vi "VelocityControl.vi"() -> ()   [LabVIEW 2024]
uses:
  <userlib>/SerialVIs/subs/portX.xctl
  <vilib>/Analysis/Matrix/Numeric/Multiply/Multiply - RM,R.vi
  <vilib>/Analysis/Matrix/Numeric/Add/Add - RM,RM.vi
  <vilib>/Analysis/Matrix/NI_Matrix.lvlib
panel:
  out "angles in deg":dbl[][](array[numeric])=[[-36.014154610778625, 83.46837607802595], [-30.58893000924773, 84.11552246158425], [-25.130229737371057, 84.75431124956516], [-19.634641879547157, 85.37840761378398], [-14.099111797871014, 85.98156827076336], [-8.52099033519902, 86.55769560527041], [-2.8980785837318344, 87.10089173956699], [2.7713319119854534, 87.60551252738216], [8.488424735842507, 88.06622131808514], [14.25383121793239, 88.47804217667414], [20.067611307066525, 88.83641207225367], [25.92924379518322, 89.13723137682419], [31.83762677661892, 89.37691186368073], [37.79108891767169, 89.55242127664737], [43.78741172147553, 89.66132347232612], [49.82386252120048, 89.70181312891611], [55.89723745208451, 89.67274407360235], [62.003913178065496, 89.57365040665448], [68.13990572321374, 89.40475978812653], [74.3009344212881, 89.16699848970453], [80.48248878103452, 88.86198808146582], [86.67989599134705, 88.4920338989176], [92.88838686585272, 88.06010569607713], [99.10315824254073, 87.5698111131883], [105.31943018881677, 87.02536275434173], [111.53249678363956, 86.43153976791783], [117.73776971827958, 85.79364484548083], [123.93081443693836, 85.11745750383476], [130.10737899266636, 84.40918439844886], [136.2634161940642, 83.67540724798543], [142.3950999438779, 82.92302874692331], [148.49883691016672, 82.15921662646399], [154.5712748202658, 81.39134581430122], [160.60930872926238, 80.62693846251224], [166.610086594057, 79.87360147972578], [172.57101538925974, 79.13896113671923], [178.4897688408234, 78.43059432862572], [184.36429763607669, 77.75595618282775], [190.1928427033293, 77.12230390469071], [195.97395184977762, 76.53661705157901], [201.7064997140921, 76.0055148080184], [207.38971064375187, 75.53517127963], [213.02318376462966, 75.131230297345], [218.6069191931086, 74.79872168252136], [224.14134407370238, 74.54198131618745], [229.62733693304716, 74.36457762732287], [235.06624874699818, 74.26924721603851], [240.45991913755014, 74.25784222094941], [245.81068625614293, 74.3312917102616], [251.12138916207132, 74.48957883430128], [256.39536184764745, 74.73173476319667], [261.6364184616579, 75.05584961216476], [266.8488296977405, 75.45909971015618], [272.0372907009237, 75.93778978209922], [277.20688116485434, 76.48740796901053], [282.3630185159317, 77.1026911624394], [287.5114051948649, 77.77769791154134], [292.65797105288704, 78.50588617461314], [297.80881179498004, 79.28019340777786], [302.9701242527187, 80.09311686760488], [308.1481390877215, 80.9367924966783], [313.3490513478763, 81.8030713039308], [318.5789491549387, 82.68359269188973]]
  out "End eff positions":dbl[][](array[numeric])=[[118.80406614490178, 11.900177338584307], [116.42319949227772, 23.62061939757193], [112.8812852219431, 35.0439304341559], [108.21380153738838, 46.05570065265972], [102.46745978970496, 56.545646687002716], [95.69973332672421, 66.40870931198523], [87.97828022716507, 75.54609771369901], [79.38026604839743, 83.86627031856675], [69.99159358054067, 91.28584292437694], [59.90604735660835, 97.73041567276096], [49.22436132278885, 103.13531122901531], [38.05321863612864, 107.44621737344505], [26.50419304598421, 110.61972804610603], [14.692641750818296, 112.62377772014376], [2.73656002273502, 113.4379648139562], [-9.244591727137866, 113.05376070468404], [-21.13107740385287, 111.47460179751994], [-32.80407982330872, 108.71586306195238], [-44.14688876654819, 104.80471248894769], [-55.04607059139518, 99.77984706465875], [-65.39260739220119, 93.6911120950671], [-75.08299374682473, 86.59900703434425], [-84.02027932691303, 78.57408233451227], [-92.11504609389742, 69.69623320037363], [-99.2863094634677, 60.05389745108567], [-105.46233368329386, 49.74316590873494], [-110.58135270533705, 38.86681481268876], [-114.5921890078627, 27.53327066602801], [-117.45476409114148, 15.855518640347135], [-119.14049569333477, 3.949966194202794], [-119.63257811260391, -8.064726094224426], [-118.92614334880528, -20.06883430367364], [-117.02830207200873, -31.942769354250004], [-113.95806467155832, -43.568271506715945], [-109.74614383008078, -54.82958930814196], [-104.43464119688832, -65.6146314423135], [-98.07662180153031, -75.81608036105384], [-90.73558084823284, -85.33245707165098], [-82.48480846305218, -94.06912702708992], [-73.40665882538579, -101.93923770089913], [-63.59173090251297, -108.86457911771357], [-53.137968720377486, -114.77635934430666], [-42.14968974863139, -119.61588771454151], [-30.73655055856092, -123.33515935792494], [-19.01245943645766, -125.89733542123625], [-7.094446110466876, -127.2771142168174], [4.898500817720759, -127.4609894057506], [16.84661775178533, -126.44739224018554], [28.630559957592617, -124.24671586001286], [40.13259377494696, -120.88122067771074], [51.23777534965642, -116.38482099965765], [61.83510394431987, -110.80275422239941], [71.81863791183875, -104.19113519753225], [81.08856159876977, -96.61639965729003], [89.55219180407094, -88.15464190371051], [97.12491296022631, -78.89085325090917], [103.7310309246349, -68.91806893492374], [109.30453615579928, -58.3364323343843], [113.78976807989173, -47.25218634980559], [117.1419736030214, -35.77660264937662], [119.32775396620747, -24.024860192164837], [120.32539544815356, -12.114884979414398], [120.12508077240803, -0.1661633589935576]]
  out "Xy coords":dbl[][](array[numeric])=[[119.4004998333631, 11.980009997619378], [117.60798934094899, 23.840319695407345], [114.64037869507271, 35.462424799360754], [110.5273192803462, 46.73020107703806], [105.30990742684473, 57.53106463250436], [99.0402737891614, 67.75709680740424], [91.78106247413862, 77.30612246852291], [83.60480512165987, 86.08273090794272], [74.59319619247974, 93.999229155298], [64.83627670417677, 100.97651817694756], [54.4315345710693, 106.94488320737224], [43.482930537200836, 111.84469031606716], [32.09985943495048, 115.62698225006315], [20.3960571480289, 118.25396759861523], [8.488464200124323, 119.69939839248653], [-3.5039426761546846, 119.94883236498062], [-15.46133931546301, 118.99977725429623], [-27.2642513631705, 116.8617157053834], [-38.79474802362048, 113.55601052248971], [-49.937620385657134, 109.11569121908178], [-60.581532551982946, 103.58512399786481], [-70.62013407064156, 97.01956845835078], [-79.95312255357898, 89.48462546120636], [-88.48724586494951, 81.05558166613805], [-96.13723386563211, 71.81665729247469], [-102.82665040427374, 61.86016461857561], [-108.48865704204738, 51.28558562805948], [-113.06668088023902, 40.19857801870846], [-116.51497981795089, 28.709919505677735], [-118.79909959205348, 16.934400967183908], [-119.89621803279354, 4.989679491994699], [-119.79537309537037, -7.00489721130977], [-118.49757238906376, -18.929483297189996], [-116.01578310953526, -30.664932243219955], [-112.37480247489547, -42.09398732275458], [-107.61100996009755, -53.10245319538249], [-101.77200380524886, -63.58033690901938], [-94.91612542972985, -73.42294691312648], [-87.11187650401664, -82.53193910207703], [-78.43723450363328, -90.81629943695152], [-68.97887358399213, -98.19325332772937], [-58.83129856088384, -104.58909268963063], [-48.095900649596956, -109.93991240993464], [-36.87994439741032, -114.19224886674193], [-25.295495931693562, -117.30361411981164], [-13.458303232206584, -119.24292043601572], [-1.4866396155469737, -119.9907909076921], [10.499878012733461, -119.5397530603009], [22.381484330708883, -117.89431351491994], [34.03946225558695, -115.07091295957667], [45.35732912555743, -111.09776187932798], [56.222000556044975, -106.01455868641854], [66.52492034149903, -99.87209306686833], [76.16314511311583, -92.73173850671873], [85.04037291495091, -84.66483906844734], [93.06790542122968, -75.75199654467893], [100.16553418069888, -66.08226511171696], [106.26234203295802, -55.752261529651356], [111.29741168928408, -44.86519977962892], [115.22043439804375, -33.529859783871714], [117.99221261311003, -21.859500512652133], [119.58505164278603, -9.970728338100312], [119.98303636600983, 2.0176680581212194]]
  out "Jacobian":dbl[][](array[numeric])=[[12.114884979414398, -46.05994356282312], [120.32539544815356, 65.41010318742471]]
  in  "Tend":dbl=6.27 format="%#_13g"
  in  "T0":dbl format="%#_13g"
  out "2D Picture":picture
  in  "picture in":picture
  out "EEVelCart":dbl[][](array[numeric])=[[3.9798472322380007, 0.0], [119.88396396221532, 0.0]]
  in  "dt":dbl=0.1 format="%#_13g"
  in  "portX":refnum<visa-resource-name>(xcontrol)="ASRL1"
  in  "L1":dbl=80.0
  in  "L2":dbl=80.0
  # "USER INPUTS"
  # "Input your equation in the Block Diagram Nodes labeled \"INPUT EQUATION\"\n(also input below for bookkeeping)"
  # "x = 3*t;\ny = 30;"
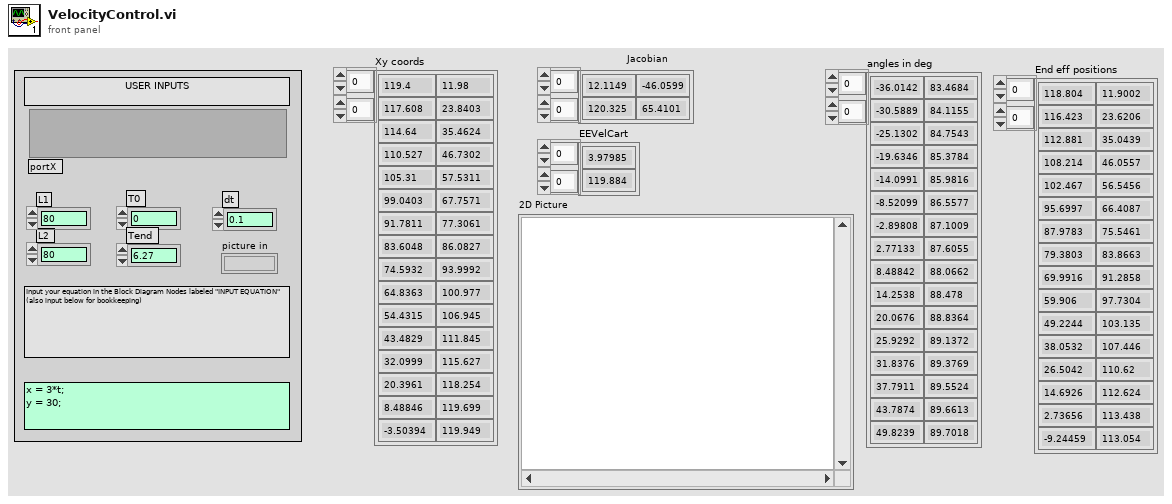
[diagram p1: front panel]
types:
  T1 = typedef "NI_Matrix.lvlib/RealMatrix.ctl" = dbl[][]
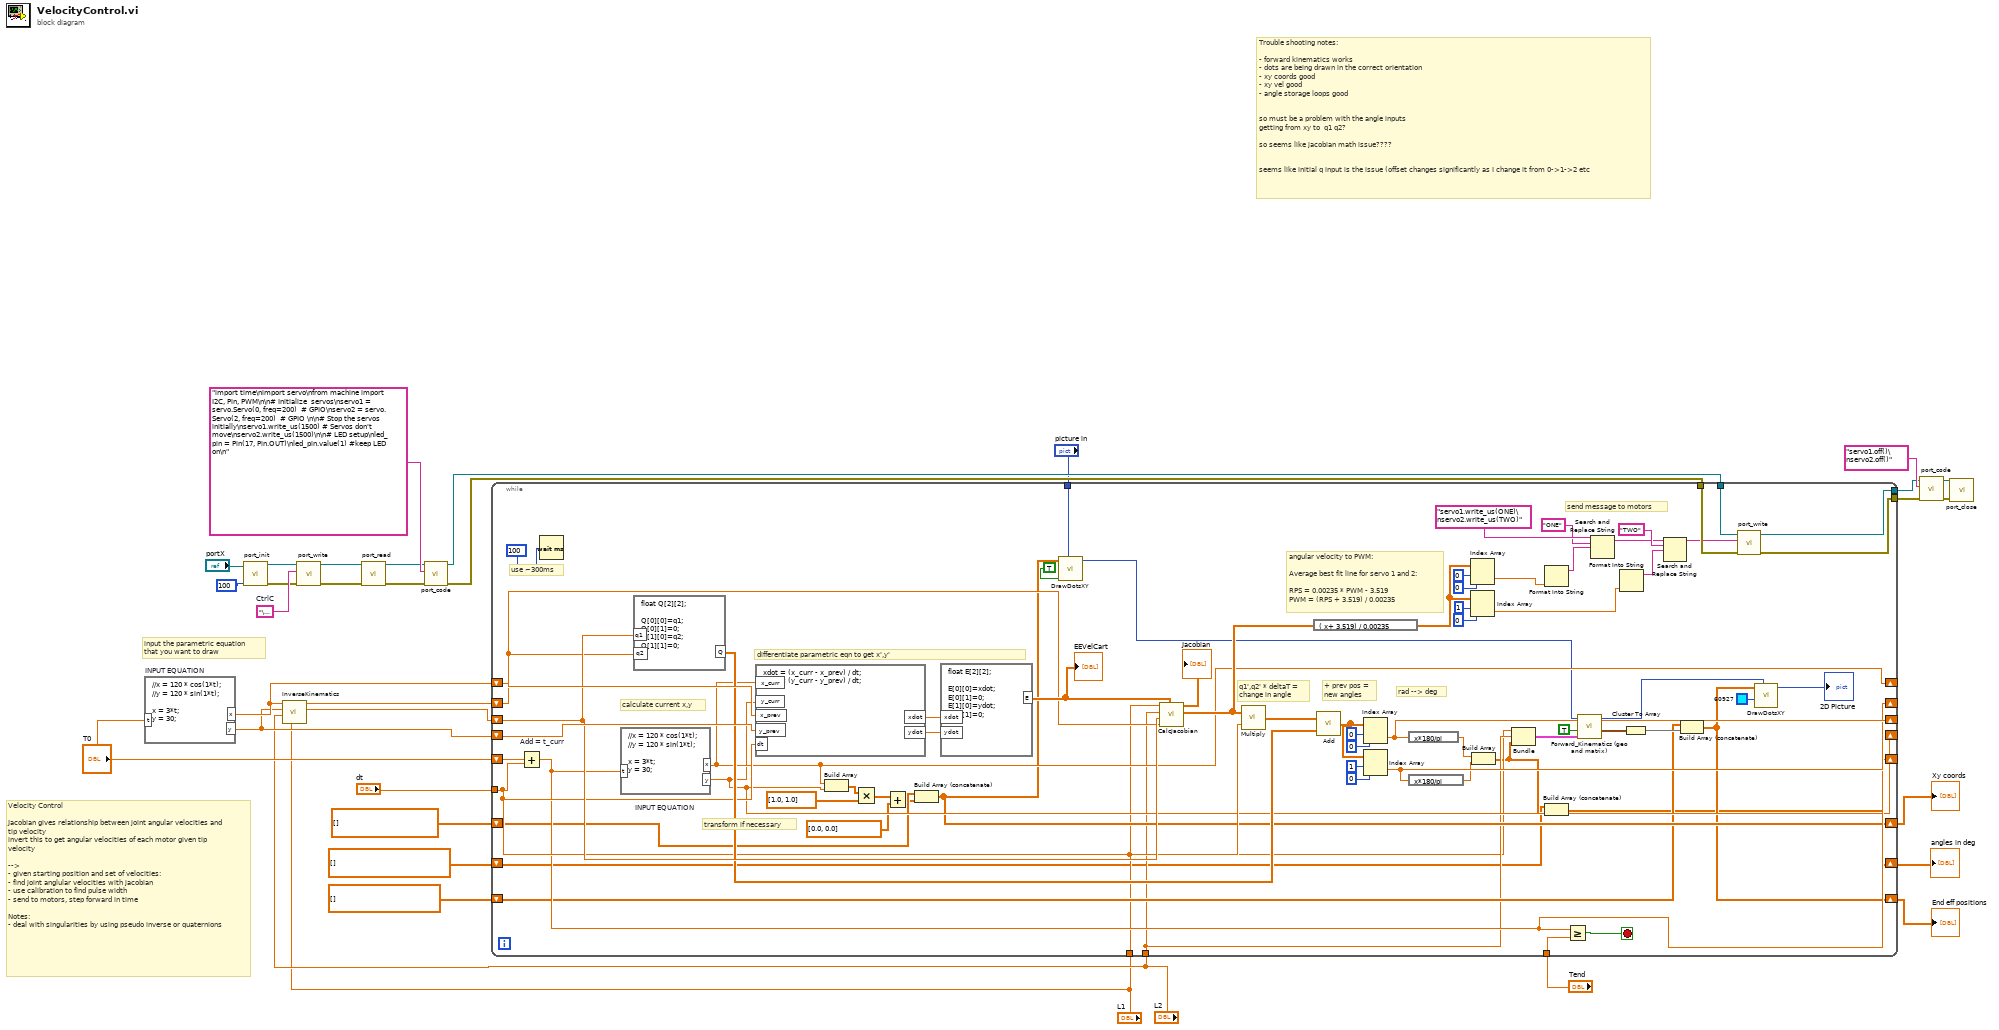
[diagram p0: block diagram]
diagram:
  w33 = "\u0003"  # CtrlC
  # "Trouble shooting notes:\n\n- forward kinematics works\n- dots are being drawn in the correct orientation\n- xy coords good\n- xy vel good\n- angle storage loops good\n\n\nso must be a problem with the angle inputs\ngetting from xy to  q1 q2?\n\nso seems like jacobian math issue???? \n\n\nseems like initial q input is the issue (offset changes significantly as I change it from 0->1->2 etc"
  # "input the parametric equation\nthat you want to draw"
  # "Velocity Control\n\nJacobian gives relationship between joint angular velocities and tip velocity\ninvert this to get angular velocities of each motor given tip velocity\n\n-->\n- given starting position and set of velocities:\n- find joint anglular velocities with jacobian\n- use calibration to find pulse width\n- send to motors, step forward in time\n\nNotes:\n- deal with singularities by using pseudo inverse or quaternions"
  n1 = formula code="//x = 120 * cos(1*t);\n//y = 120 * sin(1*t);\n\nx = 3*t;\ny = 30;" "INPUT EQUATION"("t"="T0") -> ("x"=w7:dbl, "y"=w6:dbl)
  n2 = call <userlib>:"port_init.vi"("Timeout (ms)"=u32 100, "VISA Refnum in"="portX") -> ("error out"=w32:errorcluster, "VISA Refnum out"=w24:refnum<visa-resource-name>)  [unwired: 8 in]
  n3 = call "InverseKinematics.vi"("L1"="L1", "L2"="L2", "y"=w6, "x"=w7) -> ("theta1"=w2:dbl, "theta2"=w3:dbl)  [unwired: 6 in]
  n4 = call <userlib>:"port_write.vi"("error in (no error)"=w32, "write buffer"=w33, "VISA Refnum in"=w24) -> ("error out"=w30:errorcluster, "VISA Refnum out"=w31:refnum<visa-resource-name>)  [unwired: 7 in]
  n5 = call <userlib>:"port_read.vi"("error in (no error)"=w30, "VISA Refnum in"=w31) -> ("error out"=w26:errorcluster, "VISA Refnum out"=w25:refnum<visa-resource-name>)  [unwired: 7 in, 1 out]
  n6 = call <userlib>:"port_code.vi"("error in (no error)"=w26, "Code to run"="import time\nimport servo\nfrom machine import I2C, Pin, PWM\n\n# Initialize  servos\nservo1 = servo.Servo(0, freq=200)  # GPIO\nservo2 = servo.Servo(2, freq=200)  # GPIO \n\n# Stop the servos initially\nservo1.write_us(1500) # Servos don't move\nservo2.write_us(1500)\n\n# LED setup\nled_pin = Pin(17, Pin.OUT)\nled_pin.value(1) #keep LED on\n", "VISA Refnum in"=w25) -> ("error out"=w19:errorcluster, "VISA Refnum out"=w20:refnum<visa-resource-name>)  [unwired: 7 in]
  n7 = while {
    tunnel: w20 -> [w97]
    tunnel: w19 -> [w96]
    tunnel: [w94] -> w18
    tunnel: [w93] -> w17
    tunnel: "dt" -> [w71]
    shift-right: [w67] -> _
    shift-left: w6 -> [w90]
    shift-right: [w68] -> _
    shift-left: w7 -> [w91]
    tunnel: "L2" -> [w47]
    tunnel: "L1" -> [w46]
    shift-right: [w75] -> _
    shift-left: w2 -> [w78]
    shift-right: [w74] -> _
    shift-left: w3 -> [w77]
    tunnel: "picture in" -> [w66]
    tunnel: "Tend" -> [w73]
    shift-right: [w69] -> _
    shift-left: "T0" -> [w92]
    shift-right: [w64] -> w14
    shift-left: dbl[][] [] -> [w63]
    shift-right: [w53] -> w12
    shift-left: dbl[][] [] -> [w54]
    shift-right: [w37] -> w10
    shift-left: dbl[][] [] -> [w36]
    stop <- w72 stop-if-true
    # "transform if necessary"
    # "angular velocity to PWM:\n\nAverage best fit line for servo 1 and 2:\n\nRPS = 0.00235 * PWM - 3.519\nPWM = (RPS + 3.519) / 0.00235"
    # "rad --> deg"
    # "+ prev pos =\nnew angles"
    # "q1',q2' * deltaT =\nchange in angle"
    # "calculate current x,y"
    # "differentiate parametric eqn to get x',y'"
    # "send message to motors"
    # "use ~300ms"
    n8 = Add "Add = t_curr"(x=w92, y=w71) -> (x+y=w69:dbl)
    n9 = Wait (ms)(milliseconds to wait=u32 100) -> ()  [unwired: 1 out]
    n10 = formula code="//x = 120 * cos(1*t);\n//y = 120 * sin(1*t);\n\nx = 3*t;\ny = 30;" "INPUT EQUATION"("t"=w69) -> ("x"=w68:dbl, "y"=w67:dbl)
    n11 = formula code="float Q[2][2];\n\nQ[0][0]=q1;\nQ[0][1]=0;\nQ[1][0]=q2;\nQ[1][1]=0;"("q1"=w78, "q2"=w77) -> ("Q"=w76:dbl[][])
    n12 = formula code="xdot = (x_curr - x_prev) / dt;\nydot = (y_curr - y_prev) / dt;"("x_curr"=w68, "y_curr"=w67, "x_prev"=w91, "y_prev"=w90, "dt"=w71) -> ("xdot"=w88:dbl, "ydot"=w87:dbl)
    n13 = Build Array(w68, w67) -> (w59:dbl[])
    n14 = Multiply(x=w59, y=dbl[] [1.0, 1.0]) -> (x*y=w62:dbl[])
    n15 = Add(x=w62, y=dbl[] [0.0, 0.0]) -> (x+y=w58:dbl[])
    n16 = Build Array (concatenate)(w63, w58) -> (w64:dbl[][])
    n17 = formula code="float E[2][2];\n\nE[0][0]=xdot;\nE[0][1]=0;\nE[1][0]=ydot;\nE[1][1]=0;"("xdot"=w88, "ydot"=w87) -> ("E"=w86:dbl[][])
    "EEVelCart" <- w86
    n18 = call "DrawDotsXY.vi"("Empty picture"=w66, "fill?(F)"=TRUE, "Array"=w64) -> ("2D picture"=w65:picture)  [unwired: 8 in]
    n19 = call "CalcJacobian.vi"("EndEff Velocities"=w86, "q2"=w77, "q1"=w78, "L2"=w47, "L1"=w46) -> ("Joint Angular Velocities"=w85:T1, "Jacobian"=→"Jacobian":dbl[][])  [unwired: 5 in]
    n20 = call-poly <vilib>:"Multiply.vi"("Real Scalar c"=w71, "Real Matrix A"=w85) -> ("A * c"=w89:T1)
    n21 = expression code="( x+ 3.519) / 0.00235"(w85) -> (w40:T1)
    n22 = call-poly <vilib>:"Add.vi"("Real Matrix B"=w76, "Real Matrix A"=w89) -> ("A + B"=w34:T1)
    n23 = Index Array(array=w34, index (row)=0, index (col)=0 ("disabled index (col)")) -> (element=w75:dbl)
    n24 = Index Array(array=w34, index (row)=1, index (col)=0 ("disabled index (col)")) -> (element=w74:dbl)
    n25 = expression code="x*180/pi"(w75) -> (w48:dbl)
    n26 = expression code="x*180/pi"(w74) -> (w35:dbl)
    n27 = Index Array(array=w40, index (row)=0, index (col)=0 ("disabled index (col)")) -> (element=w41:dbl)
    n28 = Index Array(array=w40, index (row)=1, index (col)=0 ("disabled index (col)")) -> (element=w39:dbl)
    n29 = Build Array(w48, w35) -> (w38:dbl[])
    n30 = Bundle("L1"=w46, "L2"=w47, w38) -> (w79:cluster{"L1":dbl, "L2":dbl, dbl[]})  [unwired: 1 in]
    n31 = Format Into String(w41) -> (resulting string=w99:string)  [unwired: 3 in, 1 out]
    n32 = Build Array (concatenate)(w36, w38) -> (w37:dbl[][])
    n33 = Greater Or Equal?(x=w69, y=w73) -> (x >= y?=w72:bool)
    n34 = call "Forward_Kinematics (geo and matrix).vi"("geometry"=w79, "geometry?"=TRUE, "picture in"=w65) -> ("end effector"=w49:cluster{"X":dbl, "Y":dbl}, "2D Picture"=w51:picture)  [unwired: 6 in, 1 out]
    n35 = Search and Replace String(input string="servo1.write_us(ONE)\nservo2.write_us(TWO)", search string="ONE", replace string=w99) -> (result string=w100:string)  [unwired: 5 in, 3 out]
    n36 = Format Into String(w39) -> (resulting string=w98:string)  [unwired: 3 in, 1 out]
    n37 = Cluster To Array(cluster=w49) -> (array=w55:dbl[])
    n38 = Search and Replace String(input string=w100, search string="TWO", replace string=w98) -> (result string=w95:string)  [unwired: 5 in, 3 out]
    n39 = Build Array (concatenate)(w54, w55) -> (w53:dbl[][])
    n40 = call <userlib>:"port_write.vi"("error in (no error)"=w96, "write buffer"=w95, "VISA Refnum in"=w97) -> ("error out"=w93:errorcluster, "VISA Refnum out"=w94:refnum<visa-resource-name>)  [unwired: 7 in]
    n41 = call "DrawDotsXY.vi"("color"=u32 60927, "Empty picture"=w51, "Array"=w53) -> ("2D picture"=→"2D Picture":picture)  [unwired: 8 in]
  }
  "Xy coords" <- w14
  "End eff positions" <- w12
  "angles in deg" <- w10
  n42 = call <userlib>:"port_code.vi"("error in (no error)"=w17, "Code to run"="servo1.off()\nservo2.off()", "VISA Refnum in"=w18) -> ("error out"=w22:errorcluster, "VISA Refnum out"=w23:refnum<visa-resource-name>)  [unwired: 7 in]
  n43 = call <userlib>:"port_close.vi"("error in (no error)"=w22, "VISA Refnum in"=w23) -> ()  [unwired: 10 in]
